vi "To XML - Empty - Returns empty element.vi"() -> ()   [LabVIEW 2013, in "JUnit XML Tests.lvlib" / "Test Suites.lvlib"]
uses:
  Test Suites.lvlib
  JUnit XML/Test Suites/Test Suites.lvclass
  <vilib>/addons/_JKI Toolkits/Caraya/classes/Assert/Assert Equal Value_Variant.vi
  <vilib>/addons/_JKI Toolkits/Caraya/classes/Test/Test.lvclass
  <vilib>/addons/_JKI Toolkits/Caraya/classes/Assert/Assert.lvclass
panel:
  out "error out":errorcluster
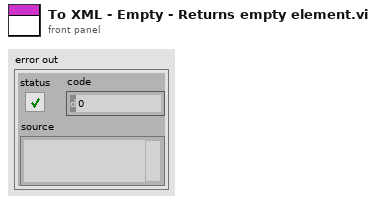
[diagram p1: front panel]
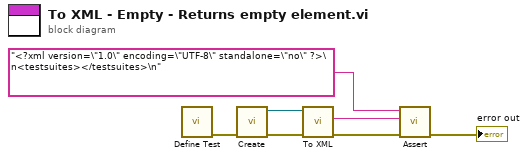
[diagram p0: block diagram]
diagram:
  n1 = call <vilib>:"Define Test.vi"() -> ("error out"=w3:errorcluster)  [unwired: 10 in, 1 out]
  n2 = call "Create.vi"("error in (no error)"=w3) -> ("error out"=w4:errorcluster, "Test Suites"=w5:refnum<class "Test Suites.lvclass">)  [unwired: 9 in]
  n3 = call-dynamic "To XML.vi"("error in (no error)"=w4, "Serializable in"=w5) -> ("error out"=w2:errorcluster, "XML"=w1:string)  [unwired: 8 in]
  n4 = call-poly <vilib>:"Assert.vi"("error in (no error)"=w2, "Actual"=w1, "Expected"="<?xml version=\"1.0\" encoding=\"UTF-8\" standalone=\"no\" ?>\n<testsuites></testsuites>\n") -> ("error out"=→"error out":errorcluster)  [unwired: 7 in, 1 out]
